vi "Global-services.vi"() -> ()   [LabVIEW 2014]
panel:
  in  "Gserver-service":refnum<vi>
  in  "HISW-service":refnum<vi>
  in  "FAMM-service":refnum<vi>
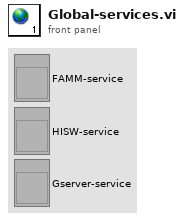
[diagram p1: front panel]
diagram:
